vi "loadActionPanel.vi"(8 "error in (no error)":errorcluster, 11 "ActionEditor in":refnum<class "ActionEditor.lvclass">) -> (0 "error out":errorcluster, 3 "ActionEditor out":refnum<class "ActionEditor.lvclass">)   [LabVIEW 2011, in "Views.lvlib" / "ScriptEditor.lvlib" / "ActionEditor.lvclass"]
uses:
  ActionEditor.lvclass
  ActionEditor.lvclass/ActionEditor.ctl
  ActionPanels/ChangeValueAction/ChangeValueAction.lvclass
  ActionPanels/ActionPanel.lvclass
  ActionPanels/RampAction/RampAction.lvclass
  ActionPanels/SingleToneAction/SingleToneAction.lvclass
  ActionPanels/SingleToneRampAction/SingleToneRampAction.lvclass
  ActionPanels/playFileAction/playFileAction.lvclass
  ActionPanels/Rf Action/rfAction.lvclass
  ActionPanels/Rf_Ramp_Action/Rf_Ramp_Action.lvclass
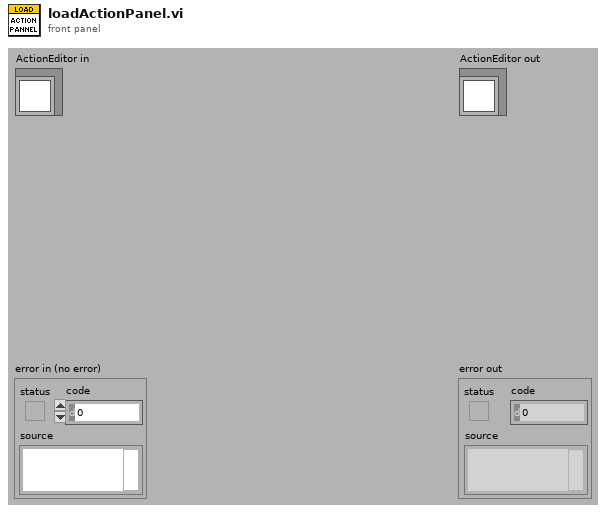
[diagram p1: front panel]
types:
  T1 = enum16{"changeValue", "pulse", "clock", "rampUp", "rampDown", "singleTone", "singleToneRamp", "playFile", "rf", "rfRamp", "delay"}
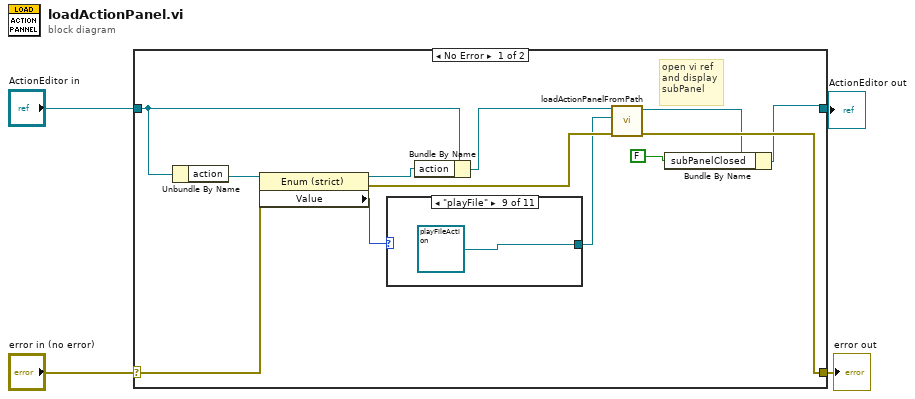
[diagram p0: block diagram]
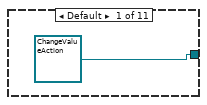
[diagram p2: hidden frame]
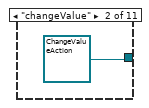
[diagram p3: hidden frame]
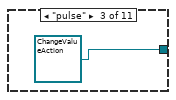
[diagram p4: hidden frame]
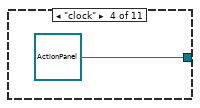
[diagram p5: hidden frame]
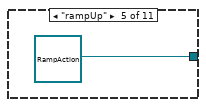
[diagram p6: hidden frame]
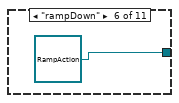
[diagram p7: hidden frame]
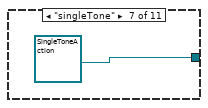
[diagram p8: hidden frame]
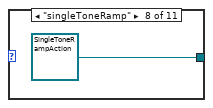
[diagram p9: hidden frame]
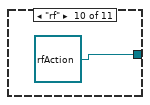
[diagram p10: hidden frame]
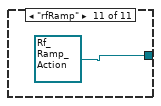
[diagram p11: hidden frame]
diagram:
  n1 = case shown="No Error" "error in (no error)" {
    selector: "error in (no error)" -> [w15 w29]
    tunnel: [w13 w29] -> w3
    tunnel: [w5 w28] -> w1
    tunnel: "ActionEditor in" -> [w10 w28]
    frame No Error {
      # "open vi ref\nand display\nsubPanel"
      n2 = Unbundle By Name(w10) -> ("action"=w16:refnum<vi>)
      n3 = property class="Enum (strict)"(reference=w16, error in=w15) -> (reference out=w11:refnum<vi>, error out=w12:errorcluster, "Value"=w14:T1)
      n4 = case shown="\"playFile\"" w14 {
        tunnel: [refnum<class "ChangeValueAction.lvclass"> refnum ("Views.lvlib:SciptEditor.lvlib:ChangeValueAction.lvclass") refnum<class "ChangeValueAction.lvclass"> refnum ("Views.lvlib:SciptEditor.lvlib:ChangeValueAction.lvclass") refnum<class "ChangeValueAction.lvclass"> refnum ("Views.lvlib:SciptEditor.lvlib:ChangeValueAction.lvclass") refnum<class "ActionPanel.lvclass"> refnum ("Views.lvlib:SciptEditor.lvlib:ActionPanel.lvclass") refnum<class "RampAction.lvclass"> refnum ("Views.lvlib:SciptEditor.lvlib:RampAction.lvclass") refnum<class "RampAction.lvclass"> refnum ("Views.lvlib:SciptEditor.lvlib:RampAction.lvclass") refnum<class "SingleToneAction.lvclass"> refnum ("Views.lvlib:SciptEditor.lvlib:SingleToneAction.lvclass") refnum<class "SingleToneRampAction.lvclass"> refnum ("Views.lvlib:SciptEditor.lvlib:SingleToneRampAction.lvclass") refnum<class "playFileAction.lvclass"> refnum ("Views.lvlib:ScriptEditor.lvlib:playFileAction.lvclass") refnum<class "rfAction.lvclass"> refnum ("Views.lvlib:ScriptEditor.lvlib:rfAction.lvclass") refnum<class "Rf_Ramp_Action.lvclass"> refnum ("Views.lvlib:ScriptEditor.lvlib:Rf_Ramp_Action.lvclass")] -> w8
        frame Default {
        }
        frame "changeValue" {
        }
        frame "pulse" {
        }
        frame "clock" {
        }
        frame "rampUp" {
        }
        frame "rampDown" {
        }
        frame "singleTone" {
        }
        frame "singleToneRamp" {
        }
        frame "playFile" {
        }
        frame "rf" {
        }
        frame "rfRamp" {
        }
      }
      n5 = Bundle By Name(cluster=w10, "action"=w11) -> (w9:refnum<class "ActionEditor.lvclass">)
      n6 = call "loadActionPanelFromPath.vi"("error in (no error)"=w12, "ActionPanel in"=w8, "ActionEditor in"=w9) -> ("error out"=w13:errorcluster, "ActionEditor out"=w6:refnum<class "ActionEditor.lvclass">)  [unwired: 7 in]
      n7 = Bundle By Name(cluster=w6, "subPanelClosed"=FALSE) -> (w5:refnum<class "ActionEditor.lvclass">)
    }
    frame Error {
    }
  }
  "error out" <- w3
  "ActionEditor out" <- w1
